vi "extract_wave_info.vi"() -> ()   [LabVIEW 2011]
panel:
  in  "Channel (0: Channel 1)":u16(ring)=1 items=["Channel 1", "Channel 2", "Channel 3", "Channel 4", "Math 1", "Math 2", "Math 3", "Math 4", "Reference 1", "Reference 2", "Reference 3", "Reference 4"]
  out "bg frames":dbl[][](graph)
  out "meas cycle array":dbl[][](array[numeric])
  out "mol TD signal":dbl[](graph)
  out "BG TD signal":dbl[](graph)
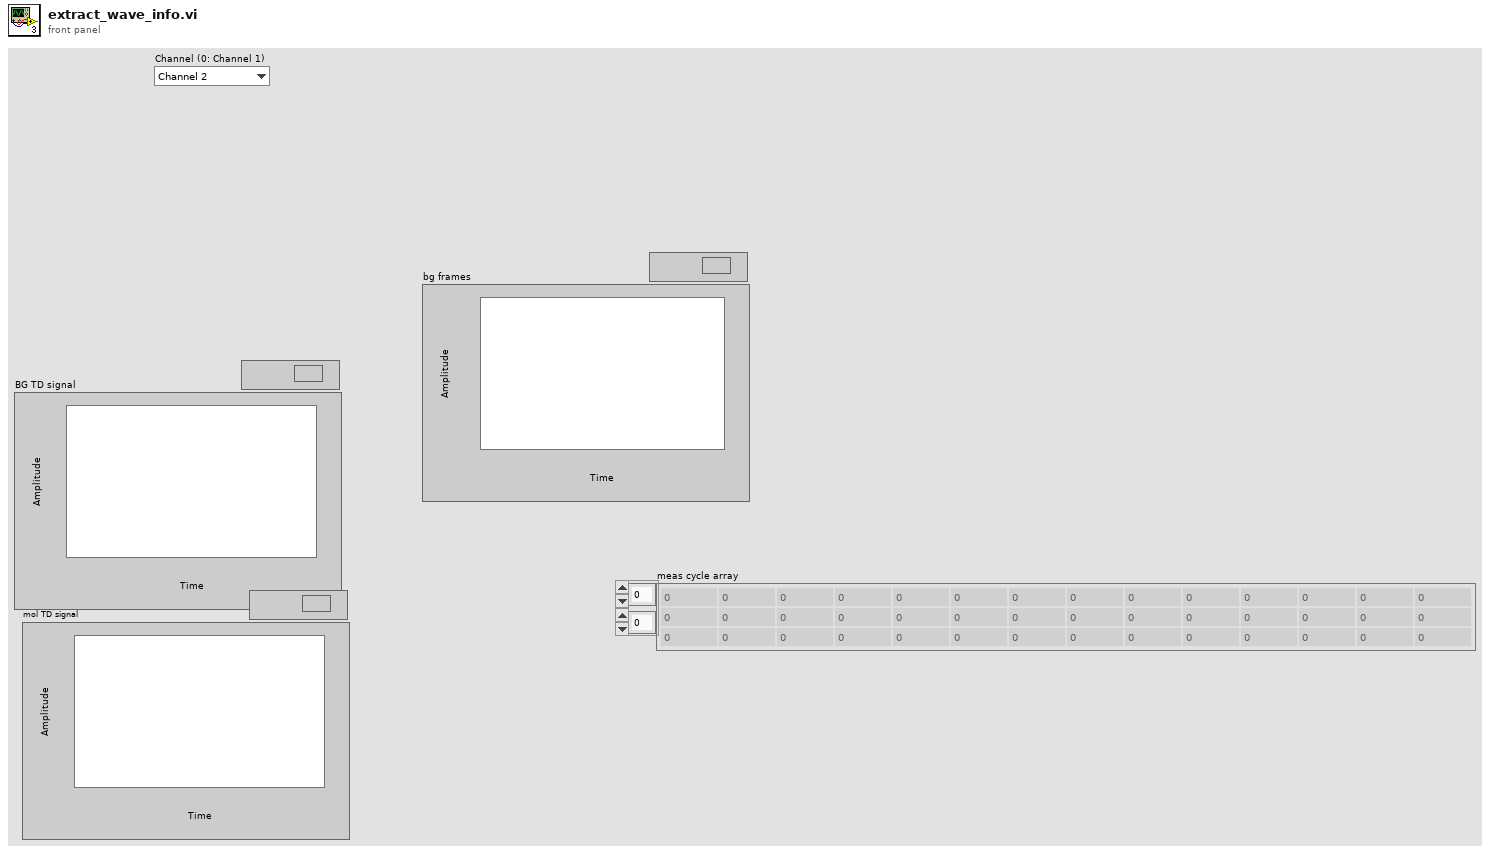
[diagram p1: front panel]
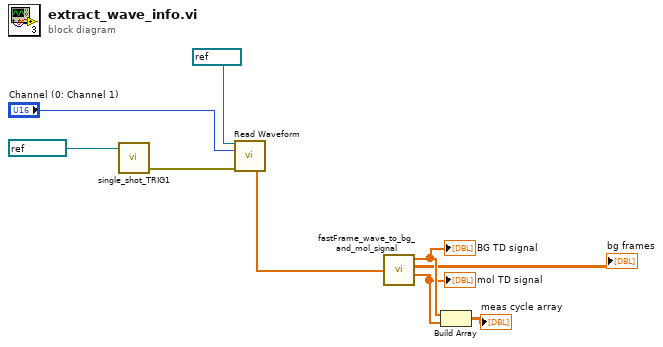
[diagram p0: block diagram]
diagram:
  n1 = call "single_shot_TRIG1.vi"("VISA resource name"=refnum<visa-resource-name> "TRIG1") -> ("error out"=w4:errorcluster)  [unwired: 3 in, 1 out]
  n2 = call "Read Waveform.vi"("VISA resource name"=refnum<visa-resource-name> "OSC", "Channel (0: Channel 1)"="Channel (0: Channel 1)", "error in (no error)"=w4) -> ("raw array data"=w1:dbl[])  [unwired: 8 in, 4 out]
  n3 = call "fastFrame_wave_to_bg_and_mol_signal.vi"("all fast frames"=w1) -> ("ave. background TD signal"=w9:dbl[], "bg frames"=→"bg frames":dbl[][], "ave. molecularTD signal"=w8:dbl[])  [unwired: 3 in]
  "BG TD signal" <- w9
  "mol TD signal" <- w8
  n4 = Build Array(w9, w8) -> (→"meas cycle array":dbl[][])
